vi "AutoVar.vi"() -> ()   [LabVIEW 2014]
panel:
  out "Scale at that point":dbl
  in  "State":string
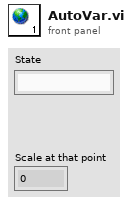
[diagram p1: front panel]
diagram:
